vi "read all bytes from serial.vi"(8 "error in (no error)":errorcluster, 11 "VISA resource name":refnum<visa-resource-name>) -> (0 "error out":errorcluster, 1 "nbytes read":i32, 2 "concatenated string":string, 3 "VISA resource name 2":refnum<visa-resource-name>)   [LabVIEW 2013]
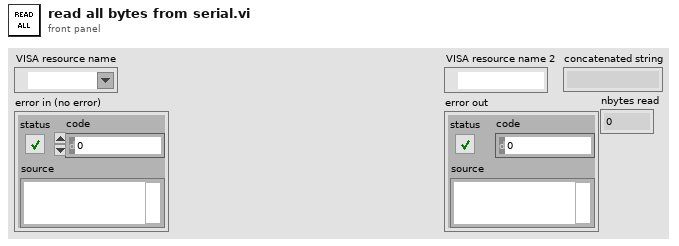
[diagram p1: front panel]
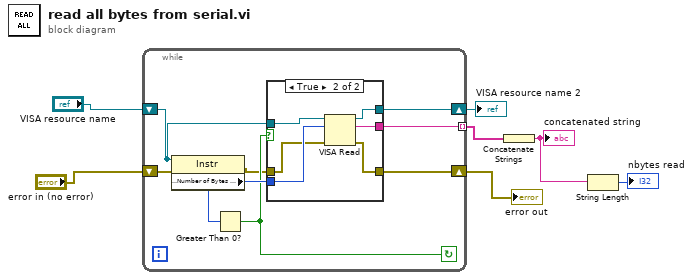
[diagram p0: block diagram]
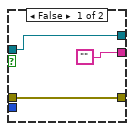
[diagram p2: hidden frame]
diagram:
  n1 = while {
    shift-right: [w14] -> w4
    shift-left: "error in (no error)" -> [w9]
    shift-right: [w13] -> w5
    shift-left: "VISA resource name" -> [w15]
    tunnel: [w12] -> w3 mode=indexing
    stop <- w10 continue-if-true
    n2 = property class="Instr"(reference=w15, error in=w9) -> (error out=w8:errorcluster, "Serial Settings:Number of Bytes at Serial Port"=w11:u32)  [unwired: 1 out]
    n3 = Greater Than 0?(x=w11) -> (x > 0?=w10:bool)
    n4 = case shown="True" w10 {
      tunnel: w15 -> [w18 w24]
      tunnel: [w16 w23] -> w14
      tunnel: [w18 w22] -> w13
      tunnel: ["" w21] -> w12
      tunnel: w11 -> [_ w20]
      tunnel: w8 -> [w16 w19]
      frame False {
      }
      frame True {
        n5 = VISA Read(VISA resource name=w24, byte count=w20, error in (no error)=w19) -> (VISA resource name out=w22:refnum<visa-resource-name>, read buffer=w21:string, error out=w23:errorcluster)  [unwired: 1 out]
      }
    }
  }
  "VISA resource name 2" <- w5
  "error out" <- w4
  n6 = Concatenate Strings(w3) -> (w2:string)
  "concatenated string" <- w2
  n7 = String Length(string=w2) -> (length=→"nbytes read":i32)
